vi "Lab_1_Mione.vi"() -> ()   [LabVIEW 2018]
panel:
  in  "operation (0:open)":T1(ring)
  in  "file path (use dialog)":path
  out "XY Graph":cluster{dbl[], dbl[]}(graph)
  out "acquiring":bool
  in  "stop acquisition":bool
  in  "Resolution":string(combo)
  in  "Averages":string(combo)
  in  "Enum":T2(ring)=enum."command"
  in  "enter":bool
  in  "stop":bool
  in  "Stop [nm]":dbl
  out "Stop [THz]":dbl
  out "Start [THz]":dbl
  in  "Start [nm]":dbl
  in  "8000/8002":bool
  out "read buffer":string
  in  "Check instruction":string
  out "Initialized":bool
  out "ID number":string
  # "Acquisition parameters"
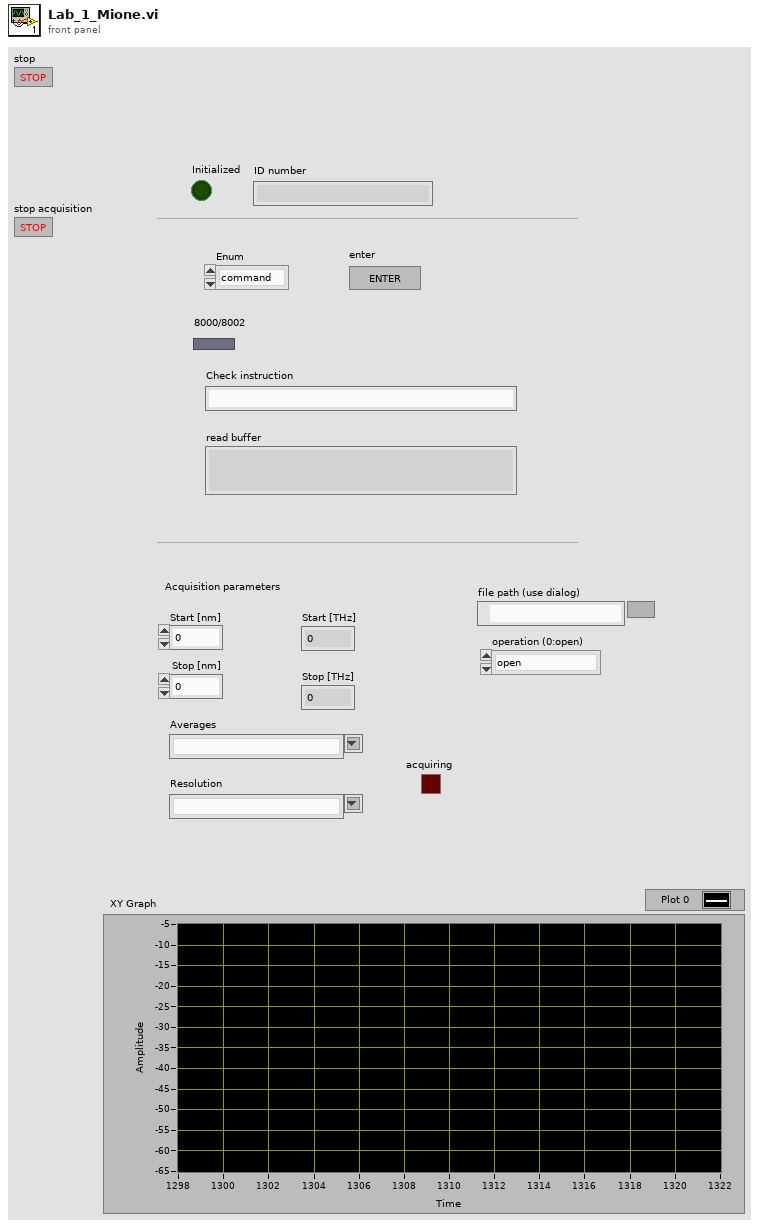
[diagram p1: front panel]
types:
  T1 = enum16{"open", "replace", "create", "open or create", "replace or create", "replace or create with confirmation"}
  T2 = enum16{"acquire", "wait", "command", "query", "initialize"}
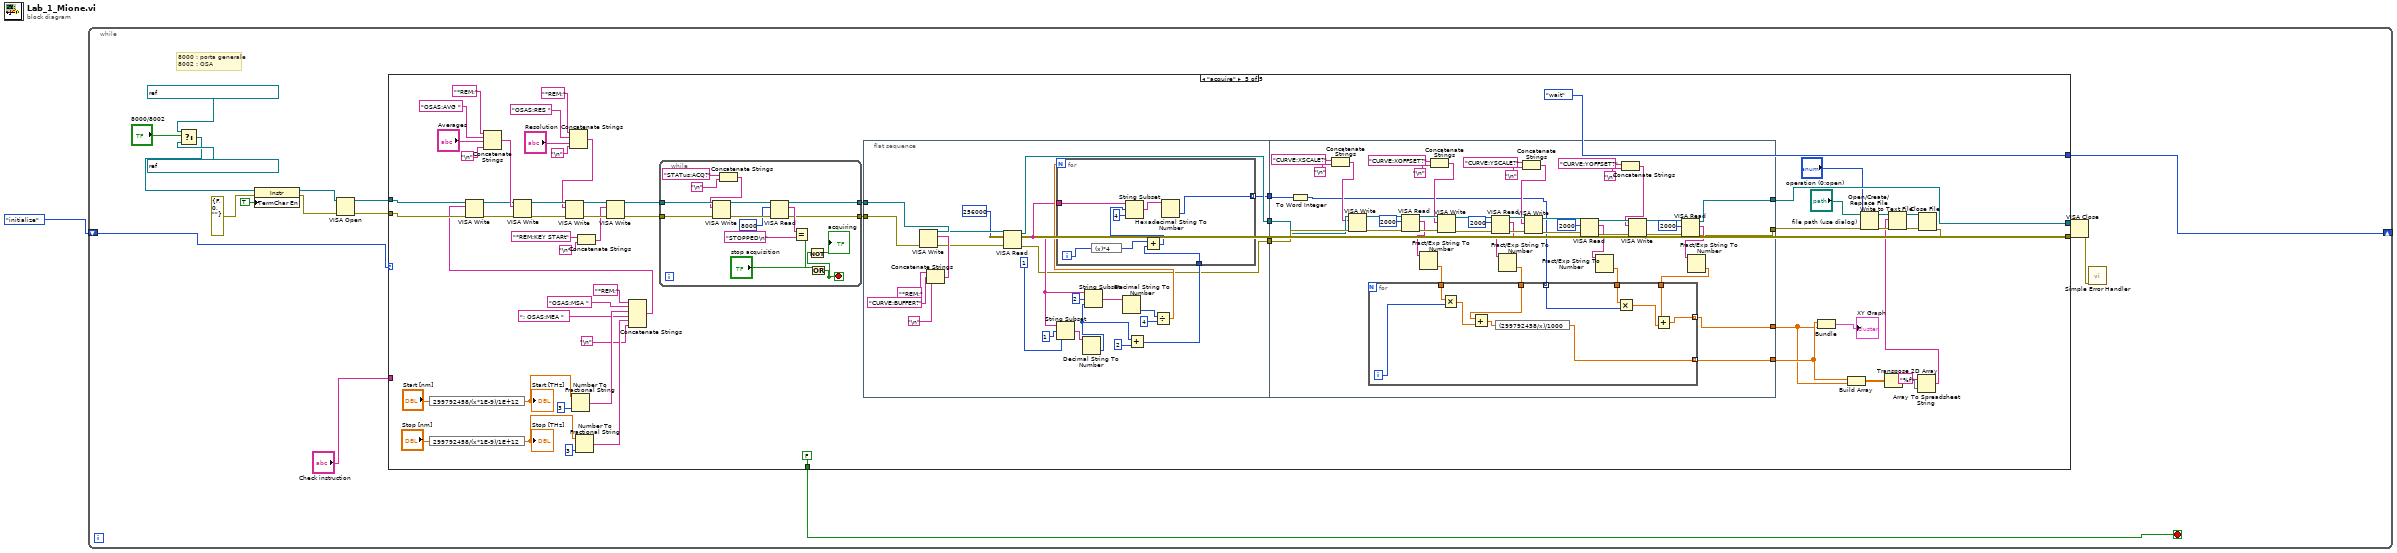
[diagram p0: block diagram]
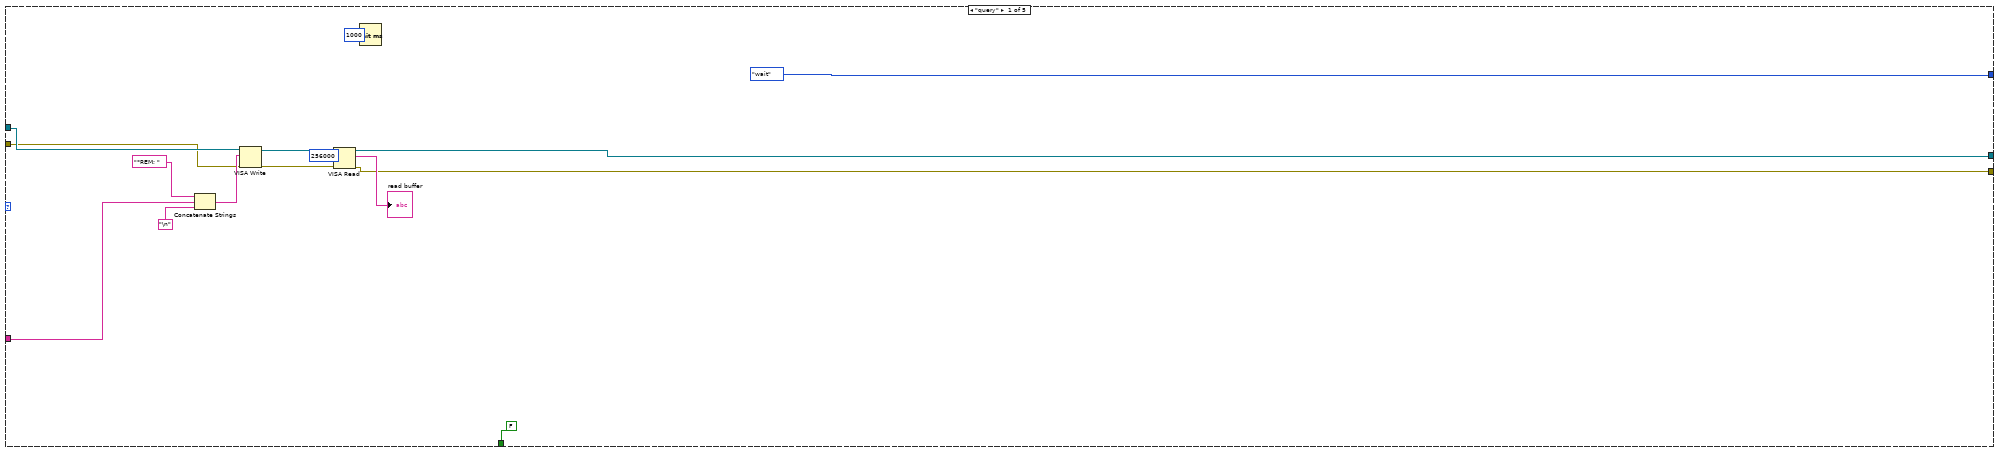
[diagram p2: hidden frame]
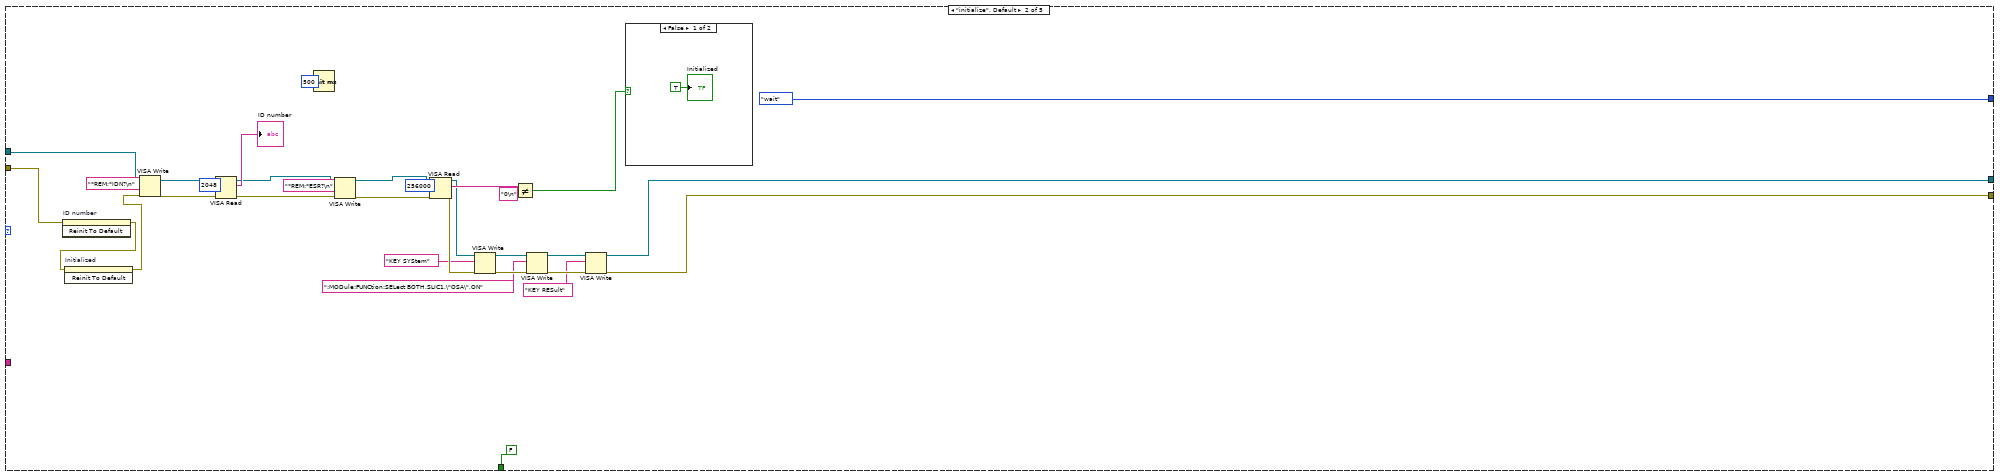
[diagram p3: hidden frame]
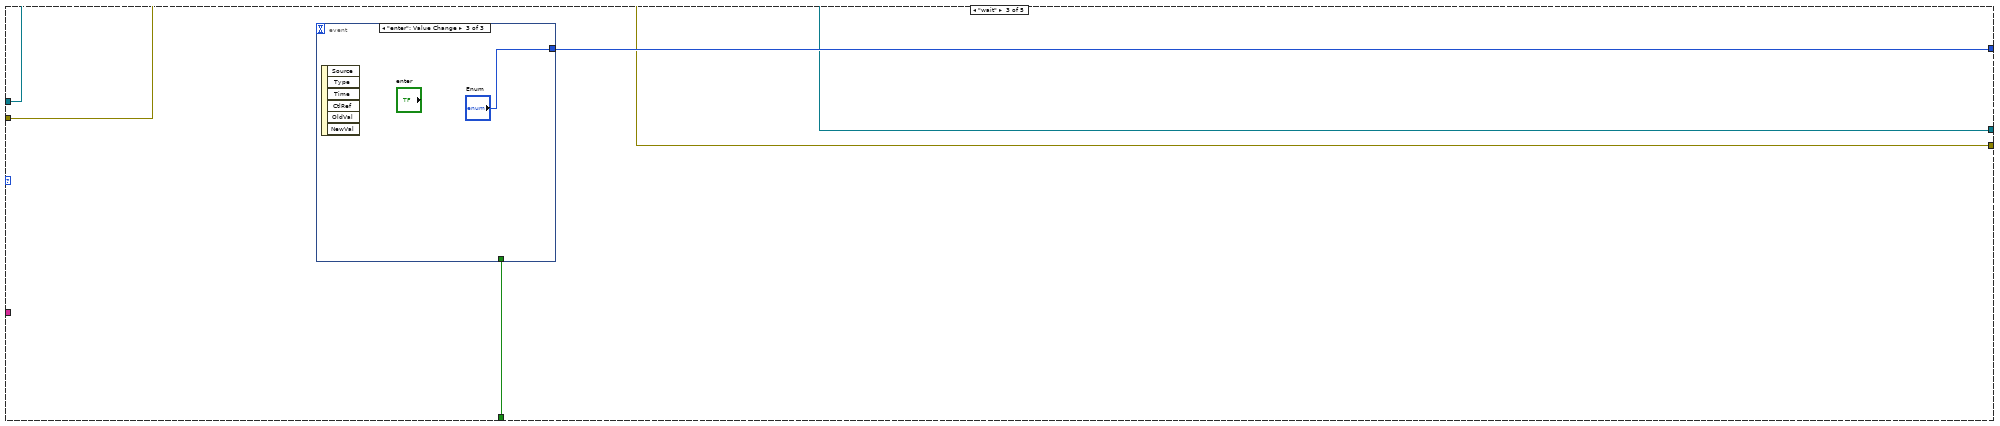
[diagram p5: hidden frame]
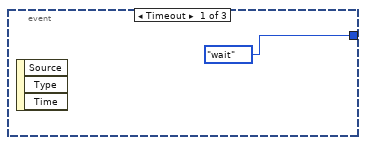
[diagram p6: hidden frame]
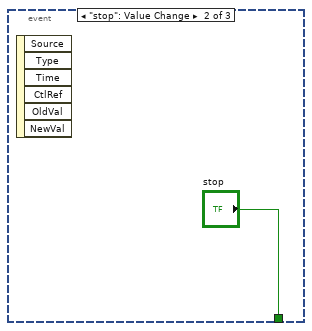
[diagram p7: hidden frame]
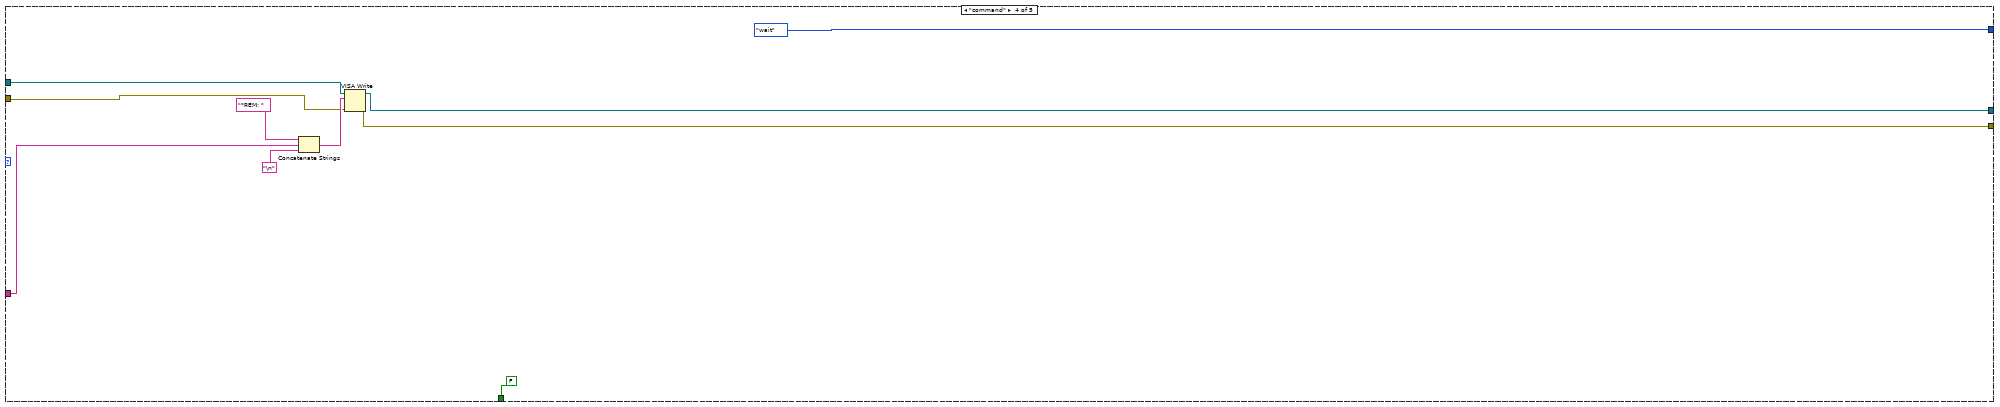
[diagram p8: hidden frame]
diagram:
  n1 = while {
    shift-right: [w9] -> _
    shift-left: T2."initialize" ("Enum") -> [w4]
    stop <- w2 stop-if-true
    # "8000 : porta generale\n8002 : OSA"
    n2 = Select(t=refnum<visa-resource-name> "TCPIP::192.168.121.192::8002::SOCKET" ("VISA resource name"), s="8000/8002", f=refnum<visa-resource-name> "TCPIP::192.168.121.192::8000::SOCKET" ("VISA resource name")) -> (s? t:f=w8:refnum<visa-resource-name>)
    n3 = property class="Instr"(reference=w8, error in=errorcluster {"status"=FALSE, "code"=0, "source"=""} ("error in (no error)"), "TermChar En"=TRUE ("Message Based Settings:Termination Character Enable")) -> (reference out=w6:refnum<visa-resource-name>, error out=w5:errorcluster)
    n4 = VISA Open(error in (no error)=w5, VISA resource name=w6) -> (VISA resource name=w17:refnum<visa-resource-name>, error out=w18:errorcluster)  [unwired: 3 in]
    n5 = case shown="\"acquire\"" w4 {
      tunnel: w18 -> [w30 w47 w67 w79 w128]
      tunnel: w17 -> [w32 w64 w68 w80 w129]
      tunnel: [w25 w35 w68 w78 w90] -> w16
      tunnel: [w24 w34 w67 w77 w86] -> w15
      tunnel: "Check instruction" -> [w21 _ _ w76 _]
      tunnel: [T2."wait" ("Enum") T2."wait" ("Enum") w69 T2."wait" ("Enum") T2."wait" ("Enum")] -> w9
      tunnel: [FALSE ("stop") FALSE ("stop") w70 FALSE ("stop") FALSE ("stop")] -> w2
      frame "query" {
        n6 = Concatenate Strings("*REM; " ("string"), w21, "\n") -> (w31:string)
        n7 = VISA Write(VISA resource name=w32, write buffer=w31, error in (no error)=w30) -> (VISA resource name out=w29:refnum<visa-resource-name>, error out=w28:errorcluster)  [unwired: 1 out]
        n8 = VISA Read(VISA resource name=w29, byte count=u32 256000, error in (no error)=w28) -> (VISA resource name out=w25:refnum<visa-resource-name>, read buffer=→"read buffer":string, error out=w24:errorcluster)  [unwired: 1 out]
        n9 = Wait (ms)(milliseconds to wait=u32 1000) -> ()  [unwired: 1 out]
      }
      frame "initialize", Default {
        n10 = invoke on="ID number" class="Str" method="Reinit To Default"(error in=w47) -> (error out=w46:errorcluster)  [unwired: 2 in, 2 out]
        n11 = invoke on="Initialized" class="Bool (strict)" method="Reinit To Default"(error in=w46) -> (error out=w45:errorcluster)  [unwired: 2 in, 2 out]
        n12 = VISA Write(VISA resource name=w64, write buffer="*REM;*IDN?\n", error in (no error)=w45) -> (VISA resource name out=w63:refnum<visa-resource-name>, error out=w62:errorcluster)  [unwired: 1 out]
        n13 = VISA Read(VISA resource name=w63, byte count=u32 2048, error in (no error)=w62) -> (VISA resource name out=w56:refnum<visa-resource-name>, read buffer=→"ID number":string, error out=w58:errorcluster)  [unwired: 1 out]
        n14 = Wait (ms)(milliseconds to wait=u32 500) -> ()  [unwired: 1 out]
        n15 = VISA Write(VISA resource name=w56, write buffer="*REM;*ESR?\n", error in (no error)=w58) -> (VISA resource name out=w53:refnum<visa-resource-name>, error out=w54:errorcluster)  [unwired: 1 out]
        n16 = VISA Read(VISA resource name=w53, byte count=u32 256000, error in (no error)=w54) -> (VISA resource name out=w44:refnum<visa-resource-name>, read buffer=w50:string, error out=w43:errorcluster)  [unwired: 1 out]
        n17 = VISA Write(VISA resource name=w44, write buffer="KEY SYStem", error in (no error)=w43) -> (VISA resource name out=w41:refnum<visa-resource-name>, error out=w40:errorcluster)  [unwired: 1 out]
        n18 = Not Equal?(x=w50, y="0\n") -> (x != y?=w51:bool)
        n19 = VISA Write(VISA resource name=w41, write buffer=":MODule:FUNCtion:SELect BOTH,SLIC1,\"OSA\",ON", error in (no error)=w40) -> (VISA resource name out=w38:refnum<visa-resource-name>, error out=w37:errorcluster)  [unwired: 1 out]
        n20 = VISA Write(VISA resource name=w38, write buffer="KEY RESult", error in (no error)=w37) -> (VISA resource name out=w35:refnum<visa-resource-name>, error out=w34:errorcluster)  [unwired: 1 out]
        n21 = case shown="False" w51 {
          frame False {
            "Initialized" <- TRUE ("Boolean")
          }
          frame True {
          }
        }
      }
      frame "wait" {
        n22 = event shown="[2] \"enter\": Value Change" {
          selector: _ -> [_ _ _]
          dyn-events: _ -> [_ _ _]
          timeout: _ -> [_ _ _]
          tunnel: [_ "stop" _] -> w70
          tunnel: [T2."wait" ("Enum") _ "Enum"] -> w69
          event Timeout {
            n23 = event-data() -> ()  [unwired: 1 in, 3 out]
          }
          event "stop": Value Change {
            n24 = event-data() -> ()  [unwired: 1 in, 6 out]
          }
          event "enter": Value Change {
            n25 = event-data() -> ()  [unwired: 1 in, 6 out]
          }
        }
      }
      frame "command" {
        n26 = Concatenate Strings("*REM; " ("string"), w76, "\n") -> (w83:string)
        n27 = VISA Write(VISA resource name=w80, write buffer=w83, error in (no error)=w79) -> (VISA resource name out=w78:refnum<visa-resource-name>, error out=w77:errorcluster)  [unwired: 1 out]
      }
      frame "acquire" {
        n28 = expression code="299792458/(x*1E-9)/1E+12"("Start [nm]") -> (w139:dbl)
        "Start [THz]" <- w139
        n29 = expression code="299792458/(x*1E-9)/1E+12"("Stop [nm]") -> (w138:dbl)
        "Stop [THz]" <- w138
        n30 = Concatenate Strings("*REM;" ("string"), "OSAS:AVG " ("string"), "Averages", "\n") -> (w123:string)
        n31 = Concatenate Strings("*REM;" ("string"), "OSAS:RES " ("string"), "Resolution", "\n") -> (w113:string)
        n32 = Number To Fractional String(number=w139, precision (6)=i16 3) -> (F-format string=w133:string)  [unwired: 2 in]
        n33 = Number To Fractional String(number=w138, precision (6)=i16 3) -> (F-format string=w131:string)  [unwired: 2 in]
        n34 = Concatenate Strings("*REM;KEY STARt", "\n") -> (w108:string)
        n35 = Concatenate Strings("*REM;" ("string"), "OSAS:MSA " ("string"), w133, "; OSAS:MEA " ("string"), w131, "\n") -> (w127:string)
        n36 = VISA Write(VISA resource name=w129, write buffer=w127, error in (no error)=w128) -> (VISA resource name out=w122:refnum<visa-resource-name>, error out=w121:errorcluster)  [unwired: 1 out]
        n37 = VISA Write(VISA resource name=w122, write buffer=w123, error in (no error)=w121) -> (VISA resource name out=w119:refnum<visa-resource-name>, error out=w120:errorcluster)  [unwired: 1 out]
        n38 = VISA Write(VISA resource name=w119, write buffer=w113, error in (no error)=w120) -> (VISA resource name out=w112:refnum<visa-resource-name>, error out=w111:errorcluster)  [unwired: 1 out]
        n39 = VISA Write(VISA resource name=w112, write buffer=w108, error in (no error)=w111) -> (VISA resource name out=w107:refnum<visa-resource-name>, error out=w106:errorcluster)  [unwired: 1 out]
        n40 = while {
          tunnel: w107 -> [w247]
          tunnel: w106 -> [w246]
          tunnel: [w236] -> w104
          tunnel: [w235] -> w105
          stop <- w232 stop-if-true
          n41 = Concatenate Strings("STATus:ACQ?", "\n") -> (w243:string)
          n42 = VISA Write(VISA resource name=w247, write buffer=w243, error in (no error)=w246) -> (VISA resource name out=w242:refnum<visa-resource-name>, error out=w241:errorcluster)  [unwired: 1 out]
          n43 = VISA Read(VISA resource name=w242, byte count=u32 8000, error in (no error)=w241) -> (VISA resource name out=w236:refnum<visa-resource-name>, read buffer=w239:string, error out=w235:errorcluster)  [unwired: 1 out]
          n44 = Equal?(x=w239, y="STOPPED\n") -> (x = y?=w234:bool)
          n45 = Or(x=w234, y="stop acquisition") -> (x .or. y?=w232:bool)
          n46 = Not(x=w232) -> (.not. x?=→"acquiring":bool)
        }
        n47 = flat-sequence {
          tunnel: w105 -> [w162]
          tunnel: w104 -> [w161]
          tunnel: [w145] -> w102
          tunnel: [w144] -> w101
          tunnel: [w143] -> w100
          tunnel: w102 -> [w219]
          tunnel: w101 -> [w220]
          tunnel: w100 -> [w176]
          tunnel: [w184] -> w90
          tunnel: [w183] -> w91
          tunnel: [w178] -> w99
          tunnel: [w177] -> w98
          frame #0 {
            n48 = Concatenate Strings("*REM;" ("string"), "CURVE:BUFFER?" ("string"), "\n") -> (w163:string)
            n49 = VISA Write(VISA resource name=w161, write buffer=w163, error in (no error)=w162) -> (VISA resource name out=w160:refnum<visa-resource-name>, error out=w159:errorcluster)  [unwired: 1 out]
            n50 = VISA Read(VISA resource name=w160, byte count=u32 256000, error in (no error)=w159) -> (VISA resource name out=w145:refnum<visa-resource-name>, read buffer=w150:string, error out=w144:errorcluster)  [unwired: 1 out]
            n51 = String Subset(string=w150, offset (0)=1, length (rest)=1 ("length (rest)")) -> (substring=w155:string)
            n52 = Decimal String To Number(string=w155) -> (number=w149:i32)  [unwired: 2 in, 1 out]
            n53 = String Subset(string=w150, offset (0)=2, length (rest)=w149) -> (substring=w154:string)
            n54 = Decimal String To Number(string=w154) -> (number=w153:i32)  [unwired: 2 in, 1 out]
            n55 = Add(x=w149, y=2) -> (x+y=w147:i32)
            n56 = Divide(x=w153, y=4) -> (x/y=w151:dbl)
            n57 = for {
              N: w151 -> [_]
              tunnel: w150 -> [w173]
              tunnel: w147 -> [w170]
              tunnel: [w167] -> w143 mode=indexing
              i -> [w172]
              n58 = expression code="(x)*4"(w172) -> (w169:i32)
              n59 = Add(x=w169, y=w170) -> (x+y=w168:i32)
              n60 = String Subset(string=w173, offset (0)=w168, length (rest)=4 ("length (rest)")) -> (substring=w171:string)
              n61 = Hexadecimal String To Number(string=w171) -> (number=w167:u32)  [unwired: 2 in, 1 out]
            }
          }
          frame #1 {
            n62 = To Word Integer(number=w176) -> (16bit integer=w175:i16[])
            n63 = Concatenate Strings("CURVE:XSCALE?" ("string"), "\n") -> (w198:string)
            n64 = VISA Write(VISA resource name=w219, write buffer=w198, error in (no error)=w220) -> (VISA resource name out=w217:refnum<visa-resource-name>, error out=w218:errorcluster)  [unwired: 1 out]
            n65 = VISA Read(VISA resource name=w217, byte count=u32 2000, error in (no error)=w218) -> (VISA resource name out=w209:refnum<visa-resource-name>, read buffer=w188:string, error out=w210:errorcluster)  [unwired: 1 out]
            n66 = Fract/Exp String To Number(string=w188) -> (number=w182:dbl)  [unwired: 3 in, 1 out]
            n67 = Concatenate Strings("CURVE:XOFFSET?" ("string"), "\n") -> (w191:string)
            n68 = VISA Write(VISA resource name=w209, write buffer=w191, error in (no error)=w210) -> (VISA resource name out=w215:refnum<visa-resource-name>, error out=w216:errorcluster)  [unwired: 1 out]
            n69 = VISA Read(VISA resource name=w215, byte count=u32 2000, error in (no error)=w216) -> (VISA resource name out=w208:refnum<visa-resource-name>, read buffer=w187:string, error out=w207:errorcluster)  [unwired: 1 out]
            n70 = Fract/Exp String To Number(string=w187) -> (number=w181:dbl)  [unwired: 3 in, 1 out]
            n71 = Concatenate Strings("CURVE:YSCALE?" ("string"), "\n") -> (w190:string)
            n72 = VISA Write(VISA resource name=w208, write buffer=w190, error in (no error)=w207) -> (VISA resource name out=w213:refnum<visa-resource-name>, error out=w214:errorcluster)  [unwired: 1 out]
            n73 = VISA Read(VISA resource name=w213, byte count=u32 2000, error in (no error)=w214) -> (VISA resource name out=w206:refnum<visa-resource-name>, read buffer=w186:string, error out=w205:errorcluster)  [unwired: 1 out]
            n74 = Fract/Exp String To Number(string=w186) -> (number=w180:dbl)  [unwired: 3 in, 1 out]
            n75 = Concatenate Strings("CURVE:YOFFSET?" ("string"), "\n") -> (w189:string)
            n76 = VISA Write(VISA resource name=w206, write buffer=w189, error in (no error)=w205) -> (VISA resource name out=w211:refnum<visa-resource-name>, error out=w212:errorcluster)  [unwired: 1 out]
            n77 = VISA Read(VISA resource name=w211, byte count=u32 2000, error in (no error)=w212) -> (VISA resource name out=w184:refnum<visa-resource-name>, read buffer=w185:string, error out=w183:errorcluster)  [unwired: 1 out]
            n78 = Fract/Exp String To Number(string=w185) -> (number=w179:dbl)  [unwired: 3 in, 1 out]
            n79 = for {
              tunnel: w182 -> [w231]
              tunnel: w181 -> [w230]
              tunnel: w180 -> [w227]
              tunnel: w179 -> [w224]
              tunnel: [w223] -> w178 mode=indexing
              tunnel: [w222] -> w177 mode=indexing
              tunnel: w175 -> [w221] mode=indexing
              i -> [w226]
              n80 = Multiply(x=w231, y=w226) -> (x*y=w229:dbl)
              n81 = Add(x=w230, y=w229) -> (x+y=w228:dbl)
              n82 = expression code="(299792458/x)/1000"(w228) -> (w223:dbl)
              n83 = Multiply(x=w227, y=w221) -> (x*y=w225:dbl)
              n84 = Add(x=w224, y=w225) -> (x+y=w222:dbl)
            }
          }
        }
        n85 = Bundle(w99, w98) -> (→"XY Graph":cluster{dbl[], dbl[]})  [unwired: 1 in]
        n86 = Build Array(w99, w98) -> (w97:dbl[][])
        n87 = Open/Create/Replace File(file path (use dialog)="file path (use dialog)", error in=w91, operation (0:open)="operation (0:open)") -> (refnum out=w93:refnum<file>, error out=w96:errorcluster)  [unwired: 3 in, 1 out]
        n88 = Transpose 2D Array(2D array=w97) -> (transposed array=w89:dbl[][])
        n89 = Array To Spreadsheet String(array=w89, 3:"%f" ("format string")) -> (spreadsheet string=w87:string)  [unwired: 1 in]
        n90 = Write to Text File(file (use dialog)=w93, text=w87, error in=w96) -> (refnum out=w94:refnum<file>, error out=w95:errorcluster)  [unwired: 1 in, 1 out]
        n91 = Close File(refnum=w94, error in=w95) -> (error out=w86:errorcluster)  [unwired: 1 out]
      }
    }
    n92 = VISA Close(VISA resource name=w16, error in (no error)=w15) -> (error out=w14:errorcluster)
    n93 = call <vilib>:"Simple Error Handler.vi"("error in (no error)"=w14) -> ()  [unwired: 4 in, 5 out]
  }
